vi "DEC_split_171213.vi"(2 "Input DEC array":sgl[][](array[numeric])) -> (1 "Channel":u32[](array[numeric]), 3 "X1":sgl[](array[numeric]), 4 "Y1":sgl[](array[numeric]), 5 "delta time":u32[](array[numeric]), 6 "ms since ON":u32[](array[numeric]), 8 "X2":sgl[](array[numeric]), 9 "Y2":sgl[](array[numeric]))   [LabVIEW 2016]
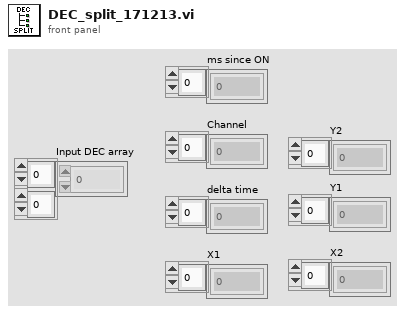
[diagram p1: front panel]
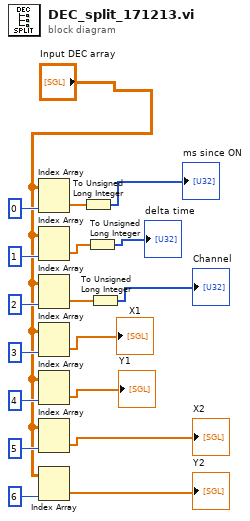
[diagram p0: block diagram]
diagram:
  n1 = Index Array(array="Input DEC array", index (col)=0 ("disabled index (col)")) -> (element=w6:sgl[])  [unwired: 1 in]
  n2 = Index Array(array="Input DEC array", index (col)=1 ("disabled index (col)")) -> (element=w4:sgl[])  [unwired: 1 in]
  n3 = Index Array(array="Input DEC array", index (col)=2 ("disabled index (col)")) -> (element=w3:sgl[])  [unwired: 1 in]
  n4 = Index Array(array="Input DEC array", index (col)=3 ("disabled index (col)")) -> (element=→"X1":sgl[])  [unwired: 1 in]
  n5 = Index Array(array="Input DEC array", index (col)=4 ("disabled index (col)")) -> (element=→"Y1":sgl[])  [unwired: 1 in]
  n6 = Index Array(array="Input DEC array", index (col)=5 ("disabled index (col)")) -> (element=→"X2":sgl[])  [unwired: 1 in]
  n7 = Index Array(array="Input DEC array", index (col)=6 ("disabled index (col)")) -> (element=→"Y2":sgl[])  [unwired: 1 in]
  n8 = To Unsigned Long Integer(number=w6) -> (unsigned 32bit integer=→"ms since ON":u32[])
  n9 = To Unsigned Long Integer(number=w4) -> (unsigned 32bit integer=→"delta time":u32[])
  n10 = To Unsigned Long Integer(number=w3) -> (unsigned 32bit integer=→"Channel":u32[])
